vi "Init.vi"(8 "error in (no error)":errorcluster, 11 "object in":refnum<class "Scope PXI CFG.lvclass">) -> (0 "error out":errorcluster, 3 "object out":refnum<class "Scope PXI CFG.lvclass">)   [LabVIEW 2023, in "Scope PXI.lvlib" / "Scope PXI CFG.lvclass"]
uses:
  Scope PXI CFG.lvclass
  Scope PXI CFG.lvclass/Scope PXI CFG.ctl
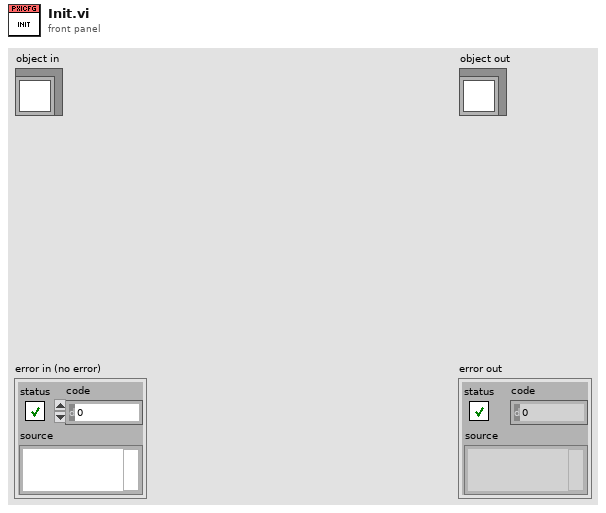
[diagram p1: front panel]
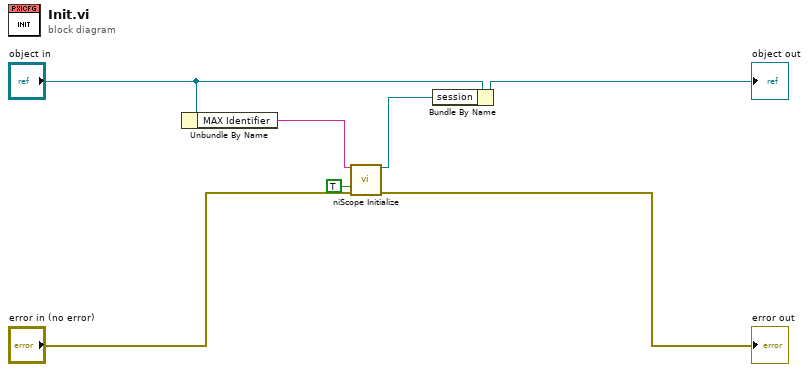
[diagram p0: block diagram]
diagram:
  n1 = Unbundle By Name("object in") -> ("MAX Identifier"=w3:string)
  n2 = call <instrlib>:"niScope Initialize.vi"("resource name"=w3, "reset device"=TRUE, "error in"="error in (no error)") -> ("instrument handle"=w2:refnum<k15>, "error out"=→"error out":errorcluster)  [unwired: 11 in]
  n3 = Bundle By Name(cluster="object in", "session"=w2) -> (→"object out":refnum<class "Scope PXI CFG.lvclass">)
